vi "TC-handler.vi"(10 "read buffer in":string) -> (3 "Thermocouple Inputs (degC)":T1)   [LabVIEW 2024]
uses:
  <vilib>/regexp/Match Regular Expression.xnode
  controls/thermocouple-input-cluster.ctl
panel:
  out "x <= y?":bool
  out "offset past match":i32
  out "concatenated string":string
  out "match + rest of string":string
  in  "search string/char (-)":string="[+-]"
  out "prototype array":dbl[](array[numeric])
  out "too big cluster":T2
  out "data array":dbl[](array[numeric])
  in  "delimiter (Tab)":string=","
  in  "format string":string
  out "substring":string
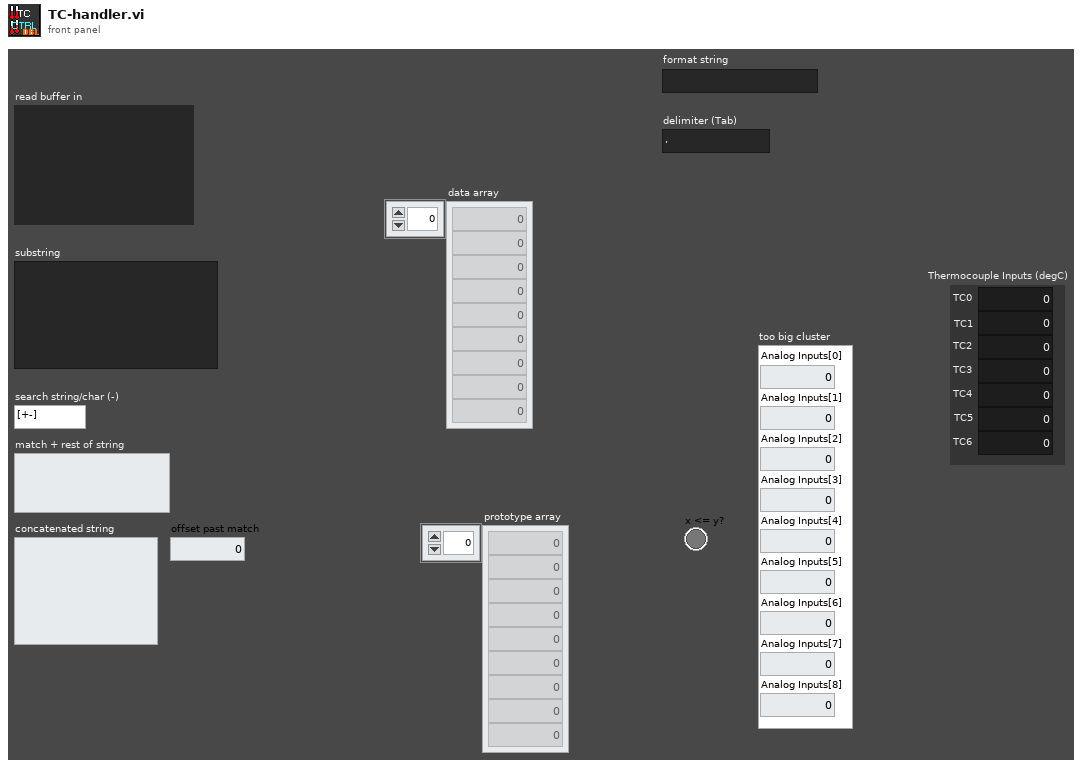
[diagram p1: front panel]
types:
  T1 = typedef "thermocouple-input-cluster.ctl" = cluster{"TC0":dbl, "TC1":dbl, "TC2":dbl, "TC3":dbl, "TC4":dbl, "TC5":dbl, "TC6":dbl}
  T2 = cluster{"Analog Inputs[0]":dbl, "Analog Inputs[1]":dbl, "Analog Inputs[2]":dbl, "Analog Inputs[3]":dbl, "Analog Inputs[4]":dbl, "Analog Inputs[5]":dbl, "Analog Inputs[6]":dbl, "Analog Inputs[7]":dbl, "Analog Inputs[8]":dbl}
  T3 = cluster{"Thermocouple Inputs (degC)[0]":dbl, "Thermocouple Inputs (degC)[1]":dbl, "Thermocouple Inputs (degC)[2]":dbl, "Thermocouple Inputs (degC)[3]":dbl, "Thermocouple Inputs (degC)[4]":dbl, "Thermocouple Inputs (degC)[5]":dbl, "Thermocouple Inputs (degC)[6]":dbl, "Thermocouple Inputs (degC)[7]":dbl, "Thermocouple Inputs (degC)[8]":dbl}
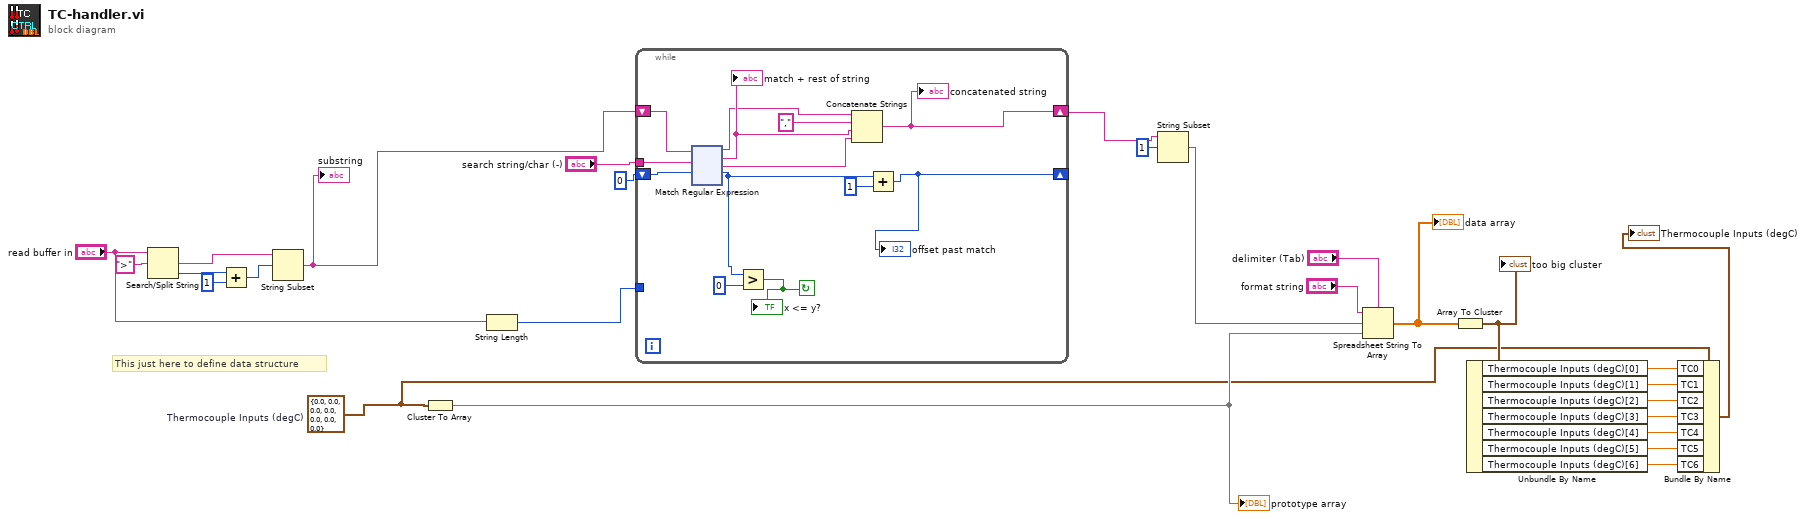
[diagram p0: block diagram]
diagram:
  w2 = T1 {"TC0"=0.0, "TC1"=0.0, "TC2"=0.0, "TC3"=0.0, "TC4"=0.0, "TC5"=0.0, "TC6"=0.0}  # Thermocouple Inputs (degC)
  # "This just here to define data structure"
  n1 = Search/Split String(string="read buffer in", search string/char (-)=">") -> (match + rest of string=w22:string, offset of match=w23:i32)  [unwired: 1 in, 1 out]
  n2 = Add(x=w23, y=1) -> (x+y=w25:i32)
  n3 = String Subset(string=w22, offset (0)=w25) -> (substring=w14:string)  [unwired: 1 in]
  "substring" <- w14
  n4 = Cluster To Array(cluster=w2) -> (array=w20:dbl[])
  "prototype array" <- w20
  n5 = String Length(string="read buffer in") -> (length=w17:i32)
  n6 = while {
    tunnel: w17 -> [_]
    tunnel: "search string/char (-)" -> [w40]
    shift-right: [w32] -> _
    shift-left: 0 ("offset past match") -> [w35]
    shift-right: [w37] -> w4
    shift-left: w14 -> [w34]
    stop <- w29 continue-if-true
    n7 = xnode ("Match Regular Expression")("input string"=w34, "regular expression"=w40, "offset (0)"=w35) -> ("before match"=w28:string, "whole match"=w39:string, "after match"=w38:string, "offset past match"=w30:i32)  [unwired: 3 in, 1 out]
    "match + rest of string" <- w39
    n8 = Greater?(x=w30, y=0) -> (0:w29:bool)
    "x <= y?" <- w29
    n9 = Concatenate Strings(w28, "," ("string"), w39, w38) -> (w37:string)
    "concatenated string" <- w37
    n10 = Add(x=w30, y=1) -> (x+y=w32:i32)
    "offset past match" <- w32
  }
  n11 = String Subset(string=w4, offset (0)=1) -> (substring=w3:string)  [unwired: 1 in]
  n12 = Spreadsheet String To Array(delimiter (Tab)="delimiter (Tab)", format string="format string", spreadsheet string=w3, array type (2D Dbl)=w20) -> (array=w19:dbl[])
  "data array" <- w19
  n13 = Array To Cluster(array=w19) -> (cluster=w13:T3)
  "too big cluster" <- w13
  n14 = Unbundle By Name(w13) -> ("Thermocouple Inputs (degC)[0]"=w12:dbl, "Thermocouple Inputs (degC)[1]"=w11:dbl, "Thermocouple Inputs (degC)[2]"=w10:dbl, "Thermocouple Inputs (degC)[3]"=w9:dbl, "Thermocouple Inputs (degC)[4]"=w8:dbl, "Thermocouple Inputs (degC)[5]"=w7:dbl, "Thermocouple Inputs (degC)[6]"=w6:dbl)
  n15 = Bundle By Name(cluster=w2, "TC0"=w12, "TC1"=w11, "TC2"=w10, "TC3"=w9, "TC4"=w8, "TC5"=w7, "TC6"=w6) -> (→"Thermocouple Inputs (degC)":T1)
